vi "CoboltLaser_EnterCurModMode.vi"(6 "ErrorIn":errorcluster, 8 "CheckResponse":bool=TRUE, 9 "ComPort":refnum<visa-resource-name>) -> (0 "ErrorOut":errorcluster, 3 "ComPortOut":refnum<visa-resource-name>)   [LabVIEW 2019]
doc: "Use this template to build a VI to use as a subVI."
panel:
  out "ResponseOK":bool
  out "Response":string
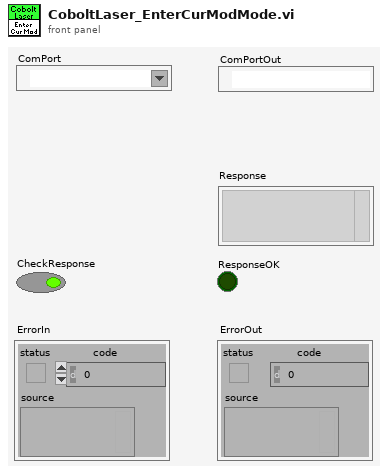
[diagram p1: front panel]
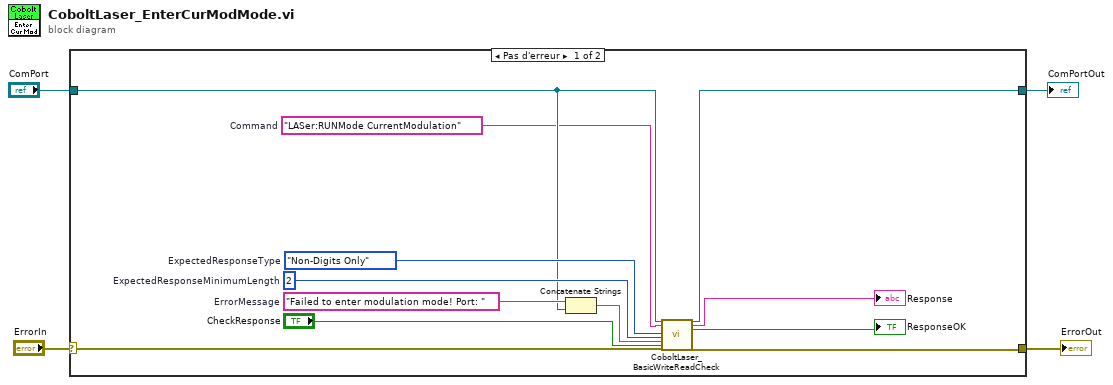
[diagram p0: block diagram]
diagram:
  n1 = case shown="Pas d'erreur" "ErrorIn" {
    selector: "ErrorIn" -> [w16 w18]
    tunnel: [w15 w18] -> w3
    tunnel: "ComPort" -> [w7 w17]
    tunnel: [w6 w17] -> w1
    frame No Error {
      w13 = 2  # ExpectedResponseMinimumLength
      w14 = enum16{"Any", "Digits Only", "Non-Digits Only"}."Non-Digits Only"  # ExpectedResponseType
      w9 = "Failed to enter modulation mode! Port: "  # ErrorMessage
      w5 = "LASer:RUNMode CurrentModulation"  # Command
      n2 = Concatenate Strings(w9, w7) -> (w8:string)
      n3 = call <userlib>:"CoboltLaser_BasicWriteReadCheck.vi"("ComPort"=w7, "Command"=w5, "ExpectedResponseType"=w14, "ExpectedResponseMinimumLength"=w13, "ErrorMessage"=w8, "GenerateError"="CheckResponse", "error in (no error)"=w16) -> ("ComPortOut"=w6:refnum<visa-resource-name>, "Response"=→"Response":string, "ResponseOK"=→"ResponseOK":bool, "error out"=w15:errorcluster)  [unwired: 17 in]
    }
    frame Error {
    }
  }
  "ErrorOut" <- w3
  "ComPortOut" <- w1
